vi "Boxcar Filter.vi"(10 "Points to average":i32, 11 "Input":dbl) -> (3 "Average":dbl format="%0.2f")   [LabVIEW 2015]
uses:
  <vilib>/Analysis/baseanly.llb/Mean (DBL).vi
  <vilib>/Analysis/NI_AALBase.lvlib
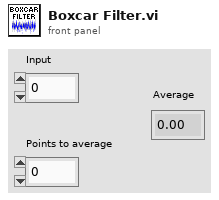
[diagram p1: front panel]
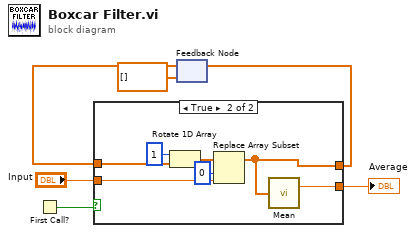
[diagram p0: block diagram]
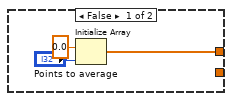
[diagram p2: hidden frame]
diagram:
  n1 = First Call?() -> (First Call?: T/F=w6:bool)
  n2 = feedback #1(dbl[] []) -> (w3:dbl[])
  n3 = case shown="True" w6 {
    tunnel: [w7 w11] -> w5
    tunnel: w3 -> [_ w13]
    tunnel: "Input" -> [_ w12]
    tunnel: [_ w10] -> w1
    frame False {
      n4 = Initialize Array(0.0 ("element"), "Points to average") -> (w7:dbl[])
    }
    frame True {
      n5 = Rotate 1D Array(1:w13, 2:1 ("n")) -> (0:w15:dbl[])
      n6 = Replace Array Subset(array=w15, new element=w12, index=0) -> (w11:dbl[])
      n7 = call-poly <vilib>:"Mean.vi"("X"=w11) -> ("mean"=w10:dbl)  [unwired: 1 out]
    }
  }
  "Average" <- w1
  n8 = feedback-in #1(w5) -> ()
